vi "Get Status.vi"(8 "error in (no error)":errorcluster, 11 "PXIe5105 in":refnum<class "PXIe5105.lvclass">) -> (0 "error out":errorcluster, 2 "Status Array (T's - OK)":bool[](array[boolean]), 3 "PXIe5105 out":refnum<class "PXIe5105.lvclass">)   [LabVIEW 2018, in "PXIe5105.lvlib" / "PXIe5105.lvclass"]
doc: "This Override method is used to get the Oscope instrument status. The status data MUST be formatted into the 'Status Array' indicator as 1D array of boolean data ."
uses:
  PXIe5105.lvclass
  PXIe5105.lvclass/PXIe5105.ctl
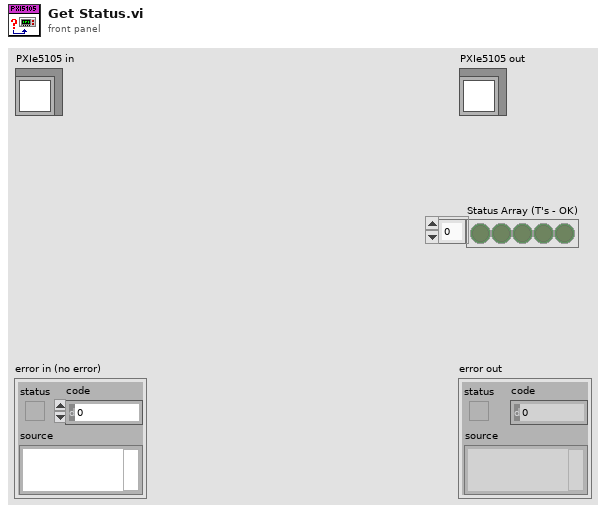
[diagram p1: front panel]
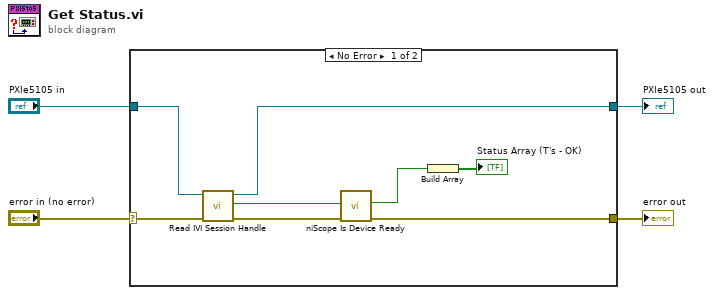
[diagram p0: block diagram]
diagram:
  n1 = case shown="No Error" "error in (no error)" {
    selector: "error in (no error)" -> [w7 w14]
    tunnel: [w12 w14] -> w3
    tunnel: [w8 w13] -> w2
    tunnel: "PXIe5105 in" -> [w9 w13]
    frame No Error {
      n2 = call "Read IVI Session Handle.vi"("error in (no error)"=w7, "PXIe5105 in"=w9) -> ("error out"=w6:errorcluster, "IVI Session Handle"=w5:refnum<k15>, "PXIe5105 out"=w8:refnum<class "PXIe5105.lvclass">)  [unwired: 7 in]
      n3 = call <instrlib>:"niScope Is Device Ready.vi"("error in"=w6, "resource name"=w5) -> ("error out"=w12:errorcluster, "Device Ready?"=w11:bool)  [unwired: 8 in]
      n4 = Build Array(w11) -> (→"Status Array (T's - OK)":bool[])
    }
    frame Error {
    }
  }
  "error out" <- w3
  "PXIe5105 out" <- w2
